vi "Pop command.vi"(8 "error in (no error)":errorcluster, 11 "File interpreter in":refnum<class "File interpreter.lvclass">) -> (0 "error out":errorcluster, 1 "Value":string, 2 "command":string, 3 "File interpreter out":refnum<class "File interpreter.lvclass">)   [LabVIEW 2018, in "File interpreter.lvclass"]
uses:
  File interpreter.lvclass
  File interpreter.lvclass/File interpreter.ctl
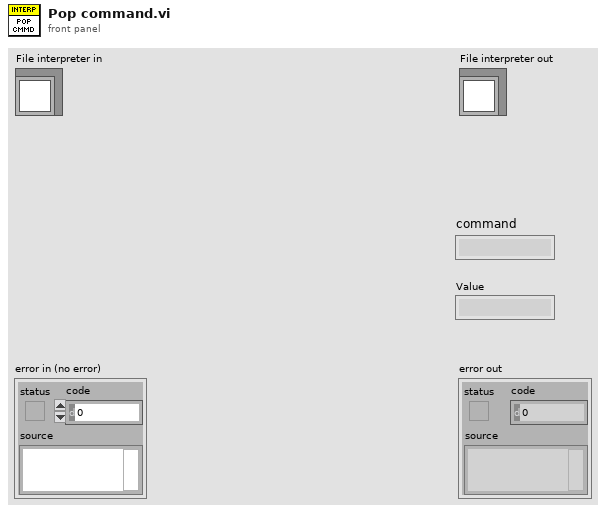
[diagram p1: front panel]
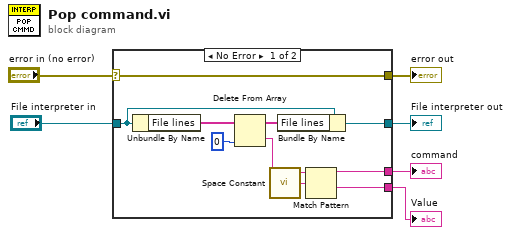
[diagram p0: block diagram]
diagram:
  n1 = case shown="No Error" "error in (no error)" {
    selector: "error in (no error)" -> [w16 w18]
    tunnel: [w16 w18] -> w5
    tunnel: [w14 w17] -> w3
    tunnel: "File interpreter in" -> [w15 w17]
    tunnel: [w9 _] -> w2
    tunnel: [w7 _] -> w1
    frame No Error {
      n2 = Unbundle By Name(w15) -> ("File lines"=w13:string[])
      n3 = Delete From Array(array=w13, index=0) -> (deleted portion=w8:string, array with subset deleted=w11:string[])  [unwired: 1 in]
      n4 = call <vilib>:"Space Constant.vi"() -> ("String"=w10:string)
      n5 = Bundle By Name(cluster=w15, "File lines"=w11) -> (w14:refnum<class "File interpreter.lvclass">)
      n6 = Match Pattern(string=w8, regular expression=w10) -> (before substring=w9:string, after substring=w7:string)  [unwired: 1 in, 2 out]
    }
    frame Error {
    }
  }
  "error out" <- w5
  "File interpreter out" <- w3
  "command" <- w2
  "Value" <- w1
